vi "Play_bottle_test.vi"(6 "Odour bottles":T4(array[cluster]), 7 "Reset counters":bool, 8 "error in (no error)":errorcluster, 9 "Test type":T1(ring), 10 "Tested channel":i32, 11 "NI cluster in":T3) -> (0 "error out":errorcluster, 3 "NI cluster out":T3, 4 "AI data":waveform(dbl)[](array[waveform]))   [LabVIEW 2016]
uses:
  NI_cluster.ctl
  <vilib>/DAQmx/write.llb/DAQmx Write (Digital 1D Wfm NChan NSamp).vi
  <vilib>/DAQmx/read.llb/DAQmx Read (Analog 1D Wfm NChan NSamp).vi
  <vilib>/Waveform/DWDTOps.llb/DWDT Uncompress Digital.vi
  <vilib>/DAQmx/miscellaneous.llb/DAQmx Fill In Error Info.vi
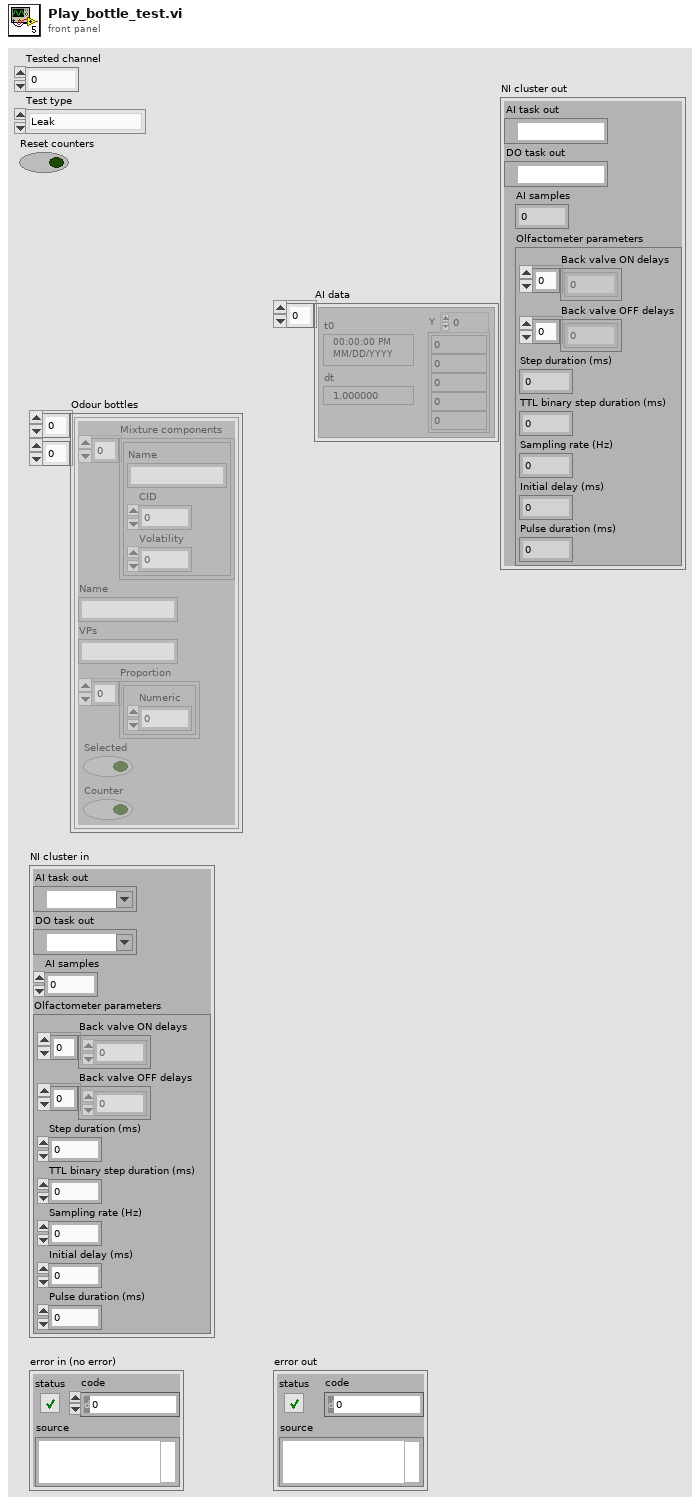
[diagram p1: front panel]
types:
  T1 = enum16{"Leak", "Flow w/o counters", "Flow w counters"}
  T2 = typedef "NI_cluster.ctl" = refnum<k21>
  T3 = cluster{"AI task out":refnum<k21>, "DO task out":T2, "AI samples":i32, "Olfactometer parameters":cluster{"Back valve ON delays":dbl[], "Back valve OFF delays":dbl[], "Step duration (ms)":dbl, "TTL binary step duration (ms)":dbl, "Sampling rate (Hz)":dbl, "Initial delay (ms)":dbl, "Pulse duration (ms)":dbl}}
  T4 = cluster{"Mixture components":cluster{"Name":string, "CID":i32, "Volatility":dbl}[], "Name":string, "VPs":string, "Proportion":cluster{"Numeric":dbl}[], "Selected":bool, "Counter":bool}[][]
  T5 = cluster{"Name":string, "Active bottles":i32[], "Concentrations":dbl[], "Unit":enum16{"%", "ppm"}}
  T6 = cluster{"Back valve ON delays":dbl[], "Back valve OFF delays":dbl[], "Step duration (ms)":dbl, "TTL binary step duration (ms)":dbl, "Sampling rate (Hz)":dbl, "Initial delay (ms)":dbl, "Pulse duration (ms)":dbl}
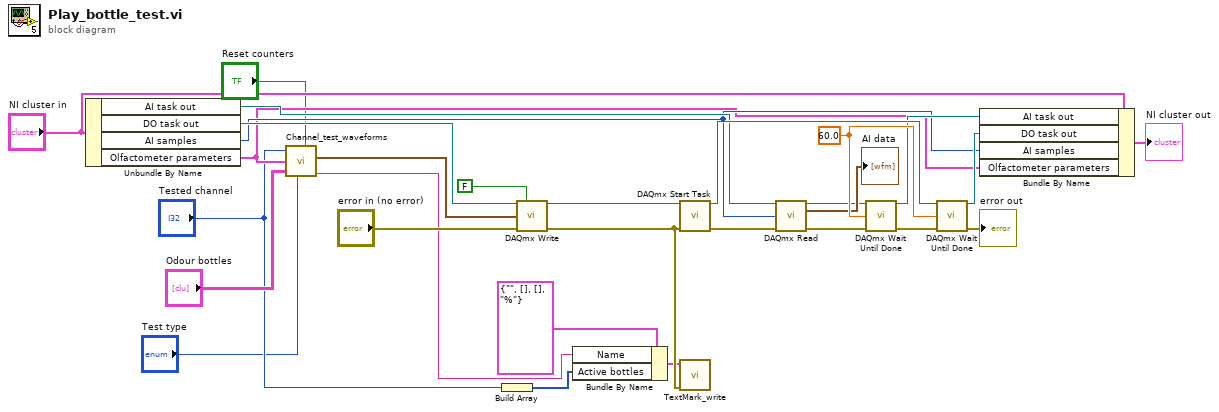
[diagram p0: block diagram]
diagram:
  w29 = 60.0 ("timeout (sec)")
  n1 = Unbundle By Name("NI cluster in") -> ("AI task out"=w18:refnum<k21>, "DO task out"=w24:T2, "AI samples"=w12:i32, "Olfactometer parameters"=w10:T6)
  n2 = call "Channel_test_waveforms.vi"("Tested channel"="Tested channel", "Olfactormeter parameters"=w10, "Odour bottles"="Odour bottles", "Test type"="Test type", "Reset counters"="Reset counters") -> ("waveform array"=w8:digitalwaveform[], "Test name"=w6:string)  [unwired: 4 in]
  n3 = Build Array("Tested channel") -> (w4:i32[])
  n4 = call-poly <vilib>:"DAQmx Write.vi"("task/channels in"=w24, "auto start"=FALSE, "data"=w8, "error in"="error in (no error)") -> ("task out"=w20:refnum<k21>, "error out"=w26:errorcluster)  [unwired: 9 in, 1 out]
  n5 = Bundle By Name(cluster=T5 {"Name"="", "Active bottles"=[], "Concentrations"=[], "Unit"=enum."%"} ("Stimulus parameters"), "Name"=w6, "Active bottles"=w4) -> (w3:T5)
  n6 = call <vilib>:"DAQmx Start Task.vi"("task/channels in"=w20, "error in"=w26) -> ("task out"=w21:refnum<k21>, "error out"=w22:errorcluster)  [unwired: 12 in]
  n7 = call "TextMark_write.vi"("error in (no error)"=w26, "Stimulus parameters"=w3) -> ()  [unwired: 10 in]
  n8 = call-poly <vilib>:"DAQmx Read.vi"("task/channels in"=w18, "number of samples per channel"=w12, "error in"=w22) -> ("task out"=w17:refnum<k21>, "data"=→"AI data":waveform(dbl)[], "error out"=w23:errorcluster)  [unwired: 10 in]
  n9 = call <vilib>:"DAQmx Wait Until Done.vi"("task/channels in"=w17, "timeout (sec)"=w29, "error in"=w23) -> ("task out"=w14:refnum<k21>, "error out"=w27:errorcluster)  [unwired: 11 in]
  n10 = call <vilib>:"DAQmx Wait Until Done.vi"("task/channels in"=w21, "timeout (sec)"=w29, "error in"=w27) -> ("task out"=w13:refnum<k21>, "error out"=→"error out":errorcluster)  [unwired: 11 in]
  n11 = Bundle By Name(cluster="NI cluster in", "AI task out"=w14, "DO task out"=w13, "AI samples"=w12, "Olfactometer parameters"=w10) -> (→"NI cluster out":T3)
